vi "CreateTopLevelDiagram.vi"(8 "error in":errorcluster, 11 "PythonConverter in":refnum<class "PythonBDConverter.lvclass">) -> (0 "error out":errorcluster, 3 "PythonConverter out":refnum<class "PythonBDConverter.lvclass">)   [LabVIEW 2014, in "PythonBDConverter.lvclass"]
uses:
  PythonBDConverter.lvclass
  PythonBDConverter.lvclass/PythonBDConverter.ctl
  VI Interpreter/Classes/TopLevelDiagram/TopLevelDiagram.lvclass
  VI Interpreter/Classes/VI Interpreter/VI Interpreter.lvclass
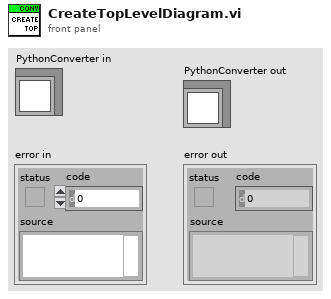
[diagram p1: front panel]
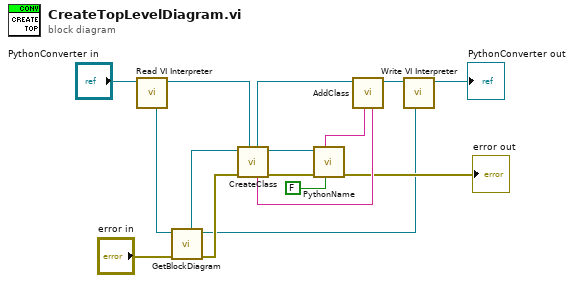
[diagram p0: block diagram]
diagram:
  n1 = call "Read VI Interpreter.vi"("PythonConverter_BD in"="PythonConverter in") -> ("PythonConverter_BD out"=w4:refnum<class "PythonBDConverter.lvclass">, "VI Interpreter"=w5:refnum<class "VI Interpreter.lvclass">)  [unwired: 7 in]
  n2 = call "GetBlockDiagram.vi"("error in"="error in", "VI Interpreter in"=w5) -> ("error out"=w10:errorcluster, "VI Interpreter out"=w1:refnum<class "VI Interpreter.lvclass">, "TopLevelDiagram"=w11:refnum<class "TopLevelDiagram.lvclass">)  [unwired: 5 in]
  n3 = call-dynamic "CreateClass.vi"("PythonConverter in"=w4, "error in"=w10, "Diagram in"=w11) -> ("error out"=w9:errorcluster, "Diagram out"=w12:refnum<class "TopLevelDiagram.lvclass">, "diagram"=w14:string, "PythonConverter out"=w13:refnum<class "PythonBDConverter.lvclass">)  [unwired: 5 in]
  n4 = call-dynamic "PythonName.vi"("add self"=FALSE, "error in"=w9, "Diagram in"=w12) -> ("error out"=→"error out":errorcluster, "UID"=w8:string)  [unwired: 5 in, 2 out]
  n5 = call "AddClass.vi"("definition"=w14, "name"=w8, "PythonConverter in"=w13) -> ("PythonConverter out"=w3:refnum<class "PythonBDConverter.lvclass">)  [unwired: 5 in, 1 out]
  n6 = call "Write VI Interpreter.vi"("VI Interpreter"=w1, "PythonConverter_BD in"=w3) -> ("PythonConverter_BD out"=→"PythonConverter out":refnum<class "PythonBDConverter.lvclass">)  [unwired: 7 in]
